vi "Get Property Folder if Exists.vi"(8 "error in (no error)":errorcluster, 9 "Property Folder Name":string, 11 "Parent ProjectItem Refnum in":refnum<vi>) -> (0 "error out":errorcluster, 1 "Folder Refnum out":refnum<vi>, 3 "Parent ProjectItem Refnum out":refnum<vi>)   [LabVIEW 2021, in "MemberVICreation.lvlib" / "BaseAccessorScripter.lvclass"]
uses:
  <resource>/Framework/Providers/LVClassLibrary/NewAccessors/BaseAccessorScripter/BaseAccessorScripter.lvclass
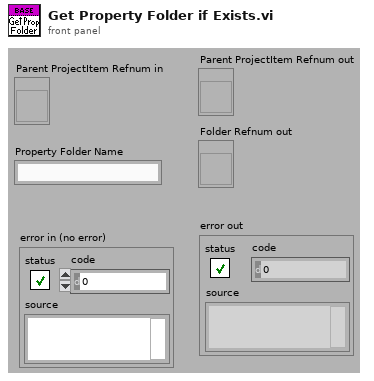
[diagram p1: front panel]
types:
  T1 = typedef "LIBUIP_item_type.ctl" = enum16{"None", "ParentLib", "Property Def Item", "VI", "Non-VI", "Folder", "Library", "Menu", "XI Ability VI", "XI Method VI", "XI Property VI", "Property Folder", "Class Private Data"}
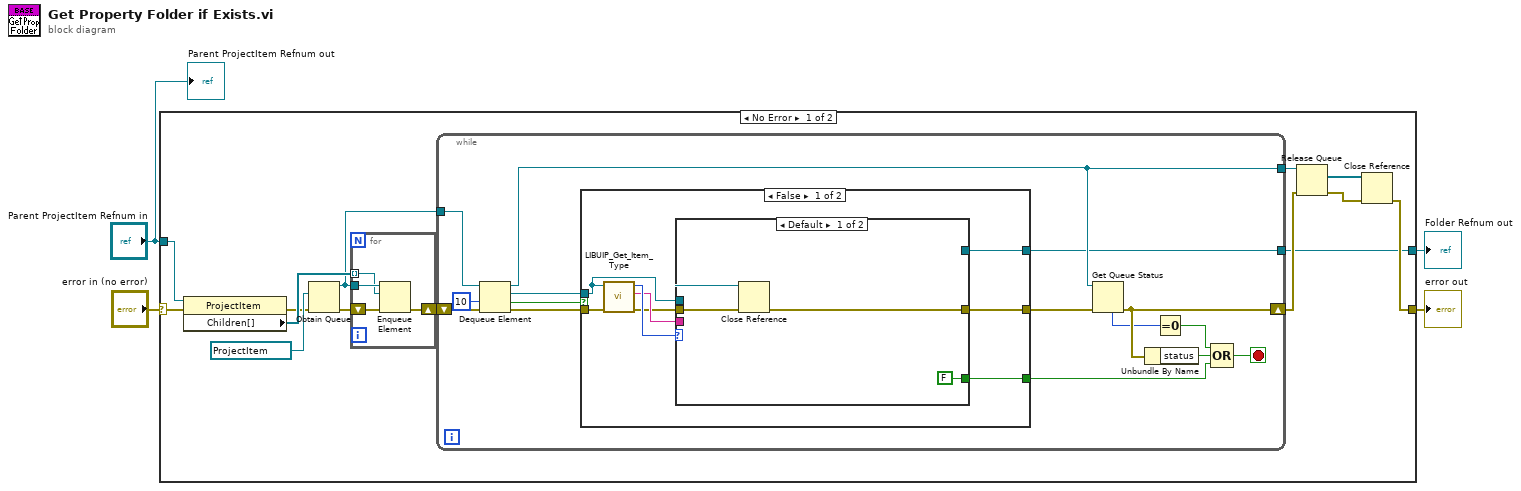
[diagram p0: block diagram]
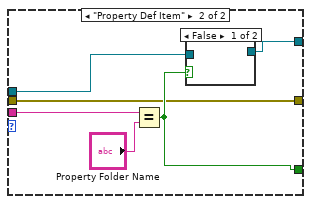
[diagram p2: hidden frame]
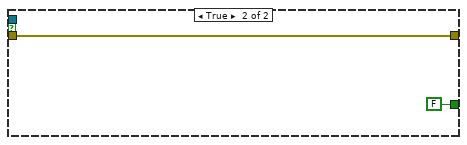
[diagram p4: hidden frame]
diagram:
  n1 = case shown="No Error" "error in (no error)" {
    selector: "error in (no error)" -> [w6 w59]
    tunnel: [w8 w59] -> w3
    tunnel: "Parent ProjectItem Refnum in" -> [w18 _]
    tunnel: [w7 _] -> w2
    frame No Error {
      n2 = property class="ProjectItem"(reference=w18, error in=w6) -> (error out=w13:errorcluster, "Children[]"=w17:refnum<vi>[])  [unwired: 1 out]
      n3 = Obtain Queue(element data type=refnum<vi> refnum ("ProjectItem Refnum"), error in (no error)=w13) -> (queue out=w5:refnum<queue>, error out=w15:errorcluster)  [unwired: 2 in, 2 out]
      n4 = for {
        tunnel: w17 -> [w21] mode=indexing
        tunnel: w5 -> [w22]
        shift-right: [w19] -> w14
        shift-left: w15 -> [w20]
        n5 = Enqueue Element(queue=w22, element=w21, error in (no error)=w20) -> (error out=w19:errorcluster)  [unwired: 3 out]
      }
      n6 = while {
        shift-right: [w30] -> w9
        shift-left: w14 -> [w37]
        tunnel: [w27] -> w12
        tunnel: [w26] -> w7
        tunnel: w5 -> [w25]
        stop <- w33 stop-if-true
        n7 = Dequeue Element(queue=w25, timeout in ms (-1)=10, error in (no error)=w37) -> (queue out=w27:refnum<queue>, element=w36:refnum<vi>, timed out?=w23:bool, error out=w35:errorcluster)
        n8 = case shown="False" w23 {
          tunnel: w36 -> [w45 _]
          tunnel: w35 -> [w44 w57]
          tunnel: [w38 FALSE] -> w34
          tunnel: [w40 w57] -> w31
          tunnel: [w39 _] -> w26
          frame False {
            n9 = call <resource>:"LIBUIP_Get_Item_Type.vi"("error in (no error)"=w44, "ProjectItem Refnum"=w45) -> ("error out"=w41:errorcluster, "Name"=w42:string, "Type"=w43:T1)  [unwired: 7 out]
            n10 = case shown="Default" w43 {
              tunnel: w42 -> [_ w54]
              tunnel: w45 -> [w49 w52]
              tunnel: w41 -> [w48 w50]
              tunnel: [w47 w50] -> w40
              tunnel: [_ w51] -> w39
              tunnel: [FALSE w53] -> w38
              frame Default {
                n11 = Close Reference(reference=w49, error in (no error)=w48) -> (error out=w47:errorcluster)
              }
              frame "Property Def Item" {
                n12 = Equal?(x=w54, y="Property Folder Name") -> (x = y?=w53:bool)
                n13 = case shown="False" w53 {
                  tunnel: w52 -> [_ w56]
                  tunnel: [_ w56] -> w51
                  frame False {
                  }
                  frame True {
                  }
                }
              }
            }
          }
          frame True {
          }
        }
        n14 = Get Queue Status(queue=w27, error in (no error)=w31) -> (error out=w30:errorcluster, # elements in queue=w29:i32)  [unwired: 7 out]
        n15 = Unbundle By Name(w30) -> ("status"=w32:bool)
        n16 = Equal To 0?(x=w29) -> (x = 0?=w28:bool)
        n17 = Compound Arithmetic op=OR(w28, w32, w34) -> (w33:bool)
      }
      n18 = Release Queue(queue=w12, error in (no error)=w9) -> (remaining elements=w11:refnum<vi>[], error out=w10:errorcluster)  [unwired: 2 out]
      n19 = Close Reference(reference=w11, error in (no error)=w10) -> (error out=w8:errorcluster)
    }
    frame Error {
    }
  }
  "error out" <- w3
  "Folder Refnum out" <- w2
  "Parent ProjectItem Refnum out" <- "Parent ProjectItem Refnum in"
